vi "test To Lower Case with Raw Name Cacher.vi"() -> ()   [LabVIEW 2017]
panel:
  out "cacher":variant
  out "Raw name 3":string
  out "Key in lower case 3":string
  out "Raw name 2":string
  out "Key in lower case 2":string
  out "Key in lower case":string
  out "Raw name":string
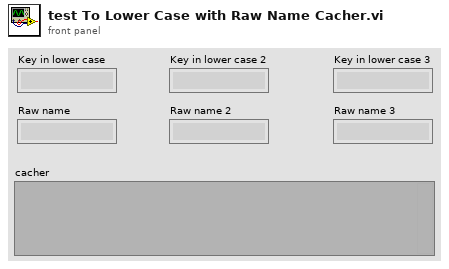
[diagram p1: front panel]
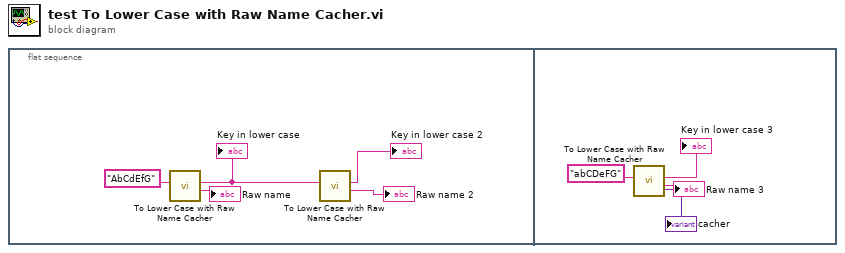
[diagram p0: block diagram]
diagram:
  n1 = flat-sequence {
    frame #0 {
      n2 = call "To Lower Case with Raw Name Cacher.vi"("key"="AbCdEfG") -> ("Raw name"=→"Raw name":string, "Key in lower case"=w3:string)  [unwired: 8 in, 1 out]
      "Key in lower case" <- w3
      n3 = call "To Lower Case with Raw Name Cacher.vi"("key"=w3) -> ("Raw name"=→"Raw name 2":string, "Key in lower case"=→"Key in lower case 2":string)  [unwired: 8 in, 1 out]
    }
    frame #1 {
      n4 = call "To Lower Case with Raw Name Cacher.vi"("key"="abCDeFG") -> ("Raw name"=→"Raw name 3":string, "Key in lower case"=→"Key in lower case 3":string, "cacher"=→"cacher":variant)  [unwired: 8 in]
    }
  }
